vi "Auto Sciscan Scope Image Delay.vi"(8 "error in":errorcluster, 9 "Auto Delay":bool=TRUE, 11 "GFG Refnum":refnum<vi>) -> (0 "error out":errorcluster, 3 "GFG Refnum Out":refnum<vi>)   [LabVIEW 2012, in "Sciscan Scope Daemon.lvlib"]
uses:
  Sciscan Scope Daemon.lvlib
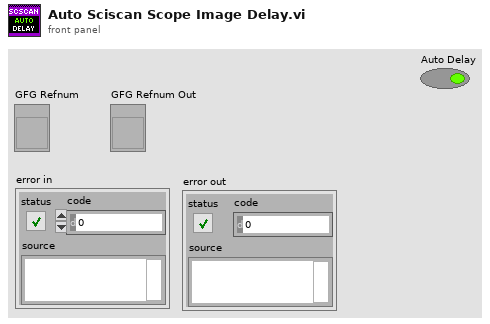
[diagram p1: front panel]
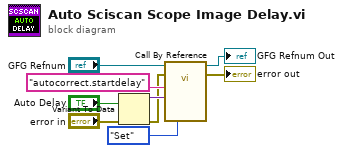
[diagram p0: block diagram]
diagram:
  n1 = Variant To Data(error in="error in", Variant="Auto Delay") -> (data=w7:variant, error out=w6:errorcluster)  [unwired: 1 in]
  n2 = call-by-ref "?"(reference="GFG Refnum", error in=w6, "Variable Name in"="autocorrect.startdelay", "Variant in"=w7, "Action"=enum16{"Init", "Set", "Get"}."Set") -> (reference out=→"GFG Refnum Out":refnum<vi>, error out=→"error out":errorcluster)  [unwired: 10 in, 7 out]
